vi "Log Data DBL.vi"(0 "TDMS Log In":refnum<class "TDMS Logger.lvclass">, 5 "Group Name":string, 7 "Channels Names":string[](array[string]), 9 "DBL Data":dbl[][](array[numeric]), 11 "Error In":errorcluster) -> (4 "TDMS Log Out":refnum<class "TDMS Logger.lvclass">, 15 "Error Out":errorcluster)   [LabVIEW 2015, in "TDMS Logger.lvlib" / "TDMS Logger.lvclass"]
doc: "Send Double data to asynch logger."
uses:
  TDMS Logger.lvclass
  TDMS Logger.lvclass/TDMS Logger.ctl
  _Typedefs/Log Action.ctl
  _Typedefs/Log Message.ctl
  _Typedefs/Data Type.ctl
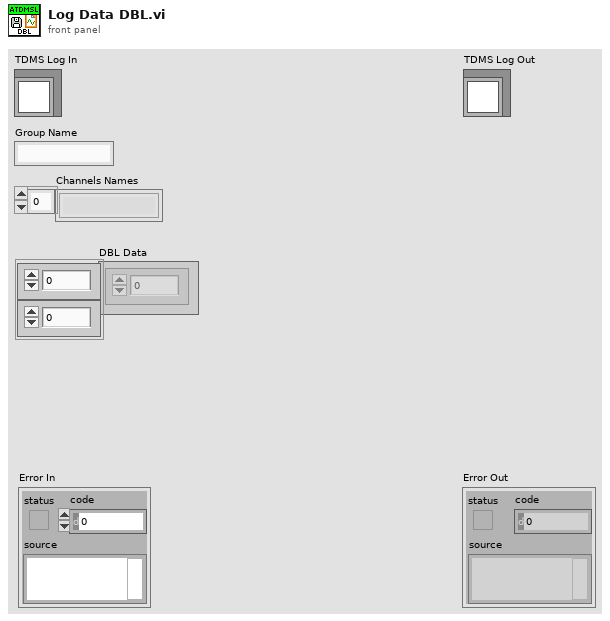
[diagram p1: front panel]
types:
  T1 = typedef "TDMS Logger.lvlib/TDMS Logger.lvclass/Data Type.ctl" = enum16{"I16", "I8", "String", "U16", "U8", "Waveform", "Double", "Single"}
  T2 = typedef "TDMS Logger.lvlib/TDMS Logger.lvclass/Log Message.ctl" = cluster{"Log Action":T3, "Variant":variant, "Data Type":T1, "Group Name":string, "Channels Names":string[]}
  T3 = typedef "TDMS Logger.lvlib/TDMS Logger.lvclass/Log Action.ctl" = enum16{"Handle Old Files", "Status Update", "Stop", "Log Data", "Initialize"}
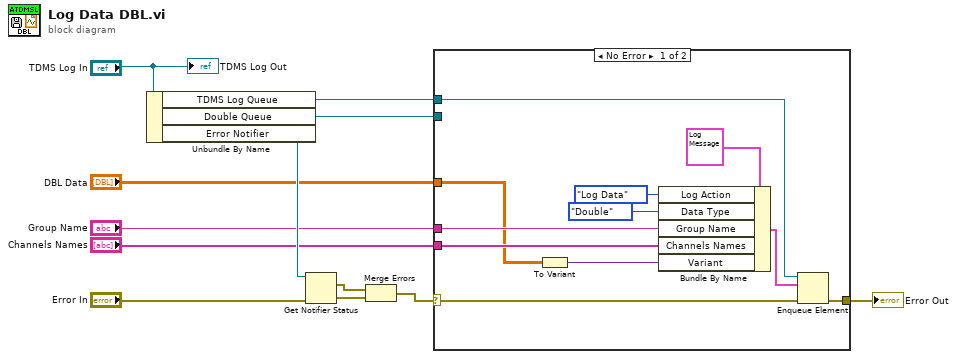
[diagram p0: block diagram]
diagram:
  n1 = Unbundle By Name("TDMS Log In") -> ("TDMS Log Queue"=w11:refnum<queue>, "Double Queue"=w1:refnum<queue>, "Error Notifier"=w8:refnum<notifier>)
  n2 = Get Notifier Status(notifier=w8, error in (no error)="Error In") -> (current notification=w5:errorcluster, error out=w6:errorcluster)  [unwired: 3 out]
  n3 = Merge Errors(w5, w6) -> (w7:errorcluster)
  n4 = case shown="No Error" w7 {
    selector: w7 -> [w15 w24]
    tunnel: [w16 w24] -> w12
    tunnel: w11 -> [w19 _]
    tunnel: "DBL Data" -> [w14 _]
    tunnel: "Group Name" -> [w17 _]
    tunnel: "Channels Names" -> [w18 _]
    tunnel: w1 -> [_ _]
    frame No Error {
      n5 = To Variant(anything=w14) -> (Variant=w13:variant)
      n6 = Bundle By Name(cluster=T2 {"Log Action"=enum."Stop", "Variant"=variant, "Data Type"=enum."String", "Group Name"="", "Channels Names"=[]} ("element"), "Log Action"=Log_Action."Log Data", "Data Type"=Data_Type."Double", "Group Name"=w17, "Channels Names"=w18, "Variant"=w13) -> (w22:T2)
      n7 = Enqueue Element(queue=w19, element=w22, error in (no error)=w15) -> (error out=w16:errorcluster)  [unwired: 1 in, 2 out]
    }
    frame Error {
    }
  }
  "Error Out" <- w12
  "TDMS Log Out" <- "TDMS Log In"
